vi "ParseMonitorRecord.vi"() -> ()   [LabVIEW 2020]
uses:
  helpers/EthFrameManagement/controls/ehternetFrame_type.ctl
  helpers/EthFrameManagement/controls/UDPFrame_type.ctl
  _controls/monitor_becw_type.ctl
  _controls/monitor_fhInfol_type.ctl
  _controls/monitor_entrySize_type.ctl
  _controls/monitor_fhw0_type.ctl
  _controls/monitor_fhw1_type.ctl
  helpers/EthFrameManagement/controls/IPFrame_type.ctl
  AIM664LV.lvlib
  helpers/EthFrameManagement/EthFrameManagement.lvlib
panel:
  out "IP header":T1
  out "IrigTime":T2
  out "FrameHeaderInfo":T3 {"FHW0"."MacID" format="%03b"}
  out "BECW":T7
  out "UDP header":T8
  out "Ethernet header":T9 {"EtherType" format="%04x"; "Src MAC" format="%02x"; "Dest MAC" format="%02x"}
  in  "QueueReadOut":T10
  out "ip src":string
  out "ip det":string
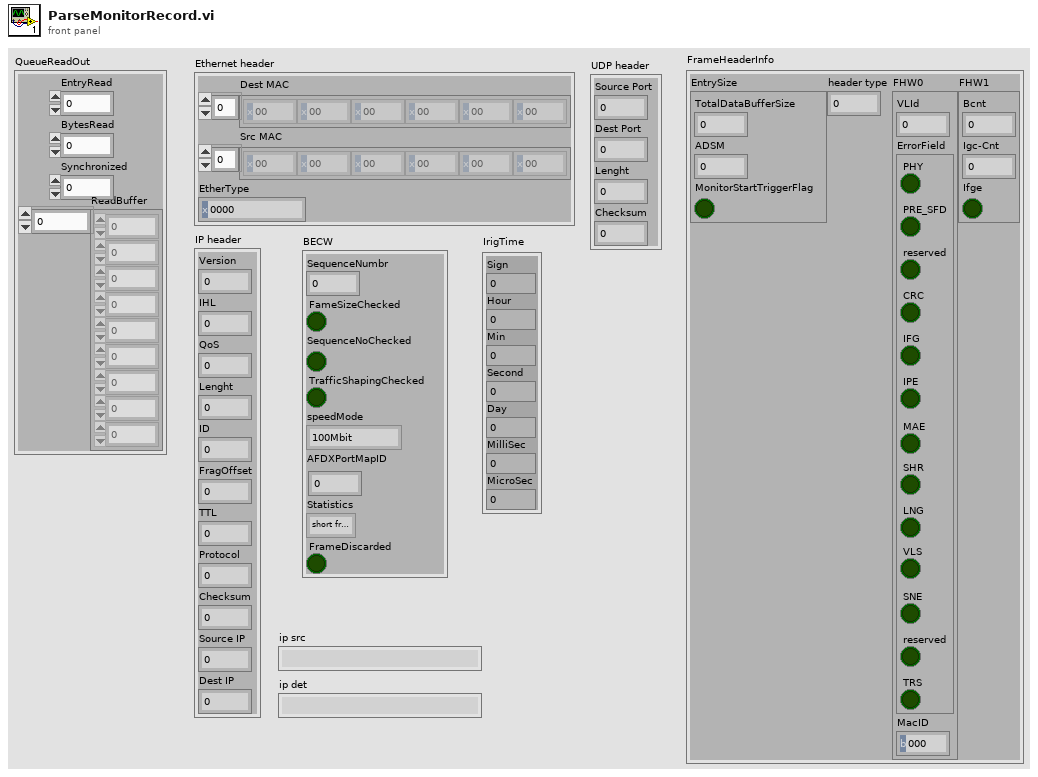
[diagram p1: front panel]
types:
  T1 = typedef "EthFrameManagement.lvlib/IPFrame_type.ctl" = cluster{"Version":u8, "IHL":u8, "QoS":u8, "Lenght":u16, "ID":u16, "FragOffset":u16, "TTL":u8, "Protocol":u8, "Checksum":u16, "Source IP":u32, "Dest IP":u32}
  T2 = cluster{"Sign":i32, "Hour":u32, "Min":u32, "Second":u32, "Day":u32, "MilliSec":u32, "MicroSec":u32}
  T3 = typedef "AIM664LV.lvlib/monitor_fhInfol_type.ctl" = cluster{"EntrySize":T4, "header type":u32, "FHW0":T5, "FHW1":T6}
  T4 = typedef "AIM664LV.lvlib/monitor_entrySize_type.ctl" = cluster{"TotalDataBufferSize":u16, "ADSM":u16, "MonitorStartTriggerFlag":bool}
  T5 = typedef "AIM664LV.lvlib/monitor_fhw0_type.ctl" = cluster{"VLId":u16, "ErrorField":cluster{"PHY":bool, "PRE_SFD":bool, "reserved":bool, "CRC":bool, "IFG":bool, "IPE":bool, "MAE":bool, "SHR":bool, "LNG":bool, "VLS":bool, "SNE":bool, "reserved":bool, "TRS":bool}, "MacID":u8}
  T6 = typedef "AIM664LV.lvlib/monitor_fhw1_type.ctl" = cluster{"Bcnt":u16, "Igc-Cnt":u16, "Ifge":bool}
  T7 = typedef "AIM664LV.lvlib/monitor_becw_type.ctl" = cluster{"SequenceNumbr":u8, "FameSizeChecked":bool, "SequenceNoChecked":bool, "TrafficShapingChecked":bool, "speedMode":enum16{"100Mbit", "10Mbit", "1Gbit"}, "AFDXPortMapID":u8, "Statistics":enum16{"short frame error 0-63Bytes", "64-127 Bytes", "128-255 Bytes", "256-511 Bytes", "512-1023 Bytes", "1024-1518 Bytes", ">1518 Bytes"}, "FrameDiscarded":bool}
  T8 = typedef "EthFrameManagement.lvlib/UDPFrame_type.ctl" = cluster{"Source Port":u16, "Dest Port":u16, "Lenght":u16, "Checksum":u16}
  T9 = typedef "EthFrameManagement.lvlib/ehternetFrame_type.ctl" = cluster{"Dest MAC":u8[], "Src MAC":u8[], "EtherType":u16}
  T10 = cluster{"EntryRead":u32, "BytesRead":u32, "Synchronized":u32, "ReadBuffer":u8[]}
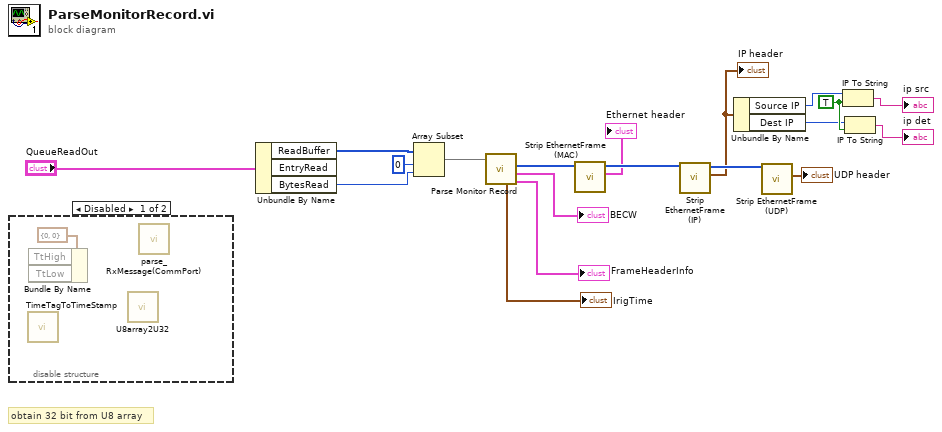
[diagram p0: block diagram]
diagram:
  w15 = TRUE ("dot notation? (F)")
  # "obtain 32 bit from U8 array"
  n1 = disable-structure shown="Disabled" {
    frame Disabled {
      n2 = call "TimeTagToTimeStamp.vi"() -> ()  [unwired: 10 in, 2 out]
      n3 = Bundle By Name(cluster=cluster{"TtHigh":u32, "TtLow":u32} {"TtHigh"=0, "TtLow"=0} ("FwIrigTime")) -> ()  [unwired: 2 in, 1 out]
      n4 = call "U8array2U32.vi"() -> ()  [unwired: 11 in, 1 out]
      n5 = call "parse_RxMessage(CommPort).vi"() -> ()  [unwired: 8 in, 4 out]
    }
    frame Enabled {
    }
  }
  n6 = Unbundle By Name("QueueReadOut") -> ("ReadBuffer"=w11:u8[], "BytesRead"=w10:u32)  [unwired: 1 out]
  n7 = Array Subset(array=w11, index=0, length=w10) -> (w4:u8[])
  n8 = call "Parse Monitor Record.vi"("Record In"=w4) -> ("FrameHeaderInfo"=→"FrameHeaderInfo":T3, "BECW"=→"BECW":T7, "Payload"=w9:u8[], "IrigTime"=→"IrigTime":T2)  [unwired: 5 in, 2 out]
  n9 = call "Strip EthernetFrame (MAC).vi"("Ethernet Frame In"=w9) -> ("Ethernet header"=→"Ethernet header":T9, "Ethernet Frame Out"=w18:u8[])  [unwired: 9 in]
  n10 = call "Strip EthernetFrame (IP).vi"("IP Frame In"=w18) -> ("IP header"=w13:T1, "IP Frame Out"=w17:u8[])  [unwired: 9 in]
  "IP header" <- w13
  n11 = Unbundle By Name(w13) -> ("Source IP"=w16:u32, "Dest IP"=w14:u32)
  n12 = call "Strip EthernetFrame (UDP).vi"("UDP Frame In"=w17) -> ("UDP header"=→"UDP header":T8)  [unwired: 9 in, 1 out]
  n13 = IP To String(1:w15, 2:w16) -> (0:→"ip src":string)
  n14 = IP To String(1:w15, 2:w14) -> (0:→"ip det":string)
